vi "UV_Parameters.vi"(6 "A/M (F:auto)":bool, 7 "R/W (F:read)":bool, 8 "error in":errorcluster, 9 "param":T1={"Time_sec"="7005.1", "Head_Pow%"=0, "Temp (C)"=50}, 10 "CHN":T2=255 items=["All"=255, "CH1"=1, "CH2"=2, "CH3"=3, "CH4"=4], 11 "VISA resource":refnum<visa-resource-name>="COM5") -> (0 "error out":errorcluster, 2 "chn param":u8[](array[numeric]) format="%.0x", 3 "VISA resource out":refnum<visa-resource-name>, 5 "Err?":bool)   [LabVIEW 2018]
uses:
  TypeDef/UVLed_channel.ctl
  TypeDef/UVLed_func.ctl
  low_level/convert/LONG_ASCII (SubVI).vi
  low_level/convert/Gen_UV_CMD (SubVI).vi
  low_level/convert/CMD_SUM (SubVI).vi
  low_level/VISA query.vi
panel:
  # "For Manual and Auto Mode Only"
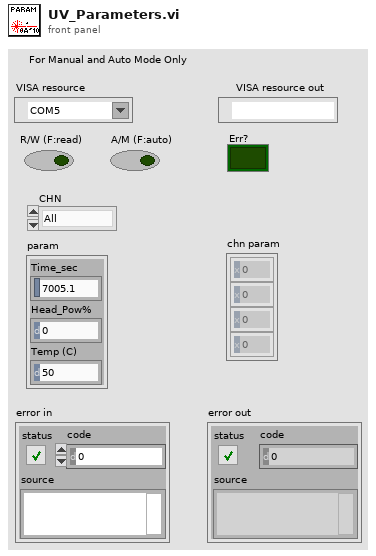
[diagram p1: front panel]
types:
  T1 = cluster{"Time_sec":string, "Head_Pow%":i32, "Temp (C)":u8}
  T2 = typedef "UVLed_channel.ctl" = u16
  T3 = typedef "UVLed_func.ctl" = u16
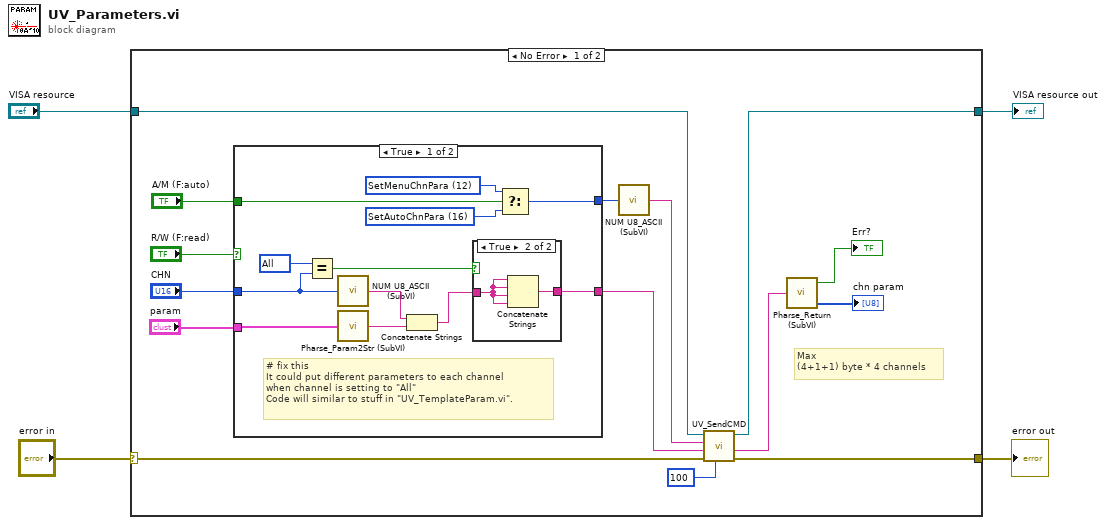
[diagram p0: block diagram]
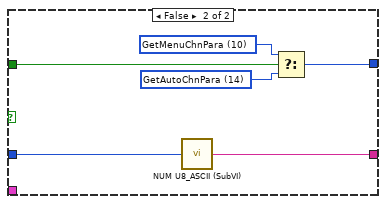
[diagram p3: hidden frame]
diagram:
  n1 = case shown="No Error" "error in" {
    selector: "error in" -> [w16 w42]
    tunnel: [w15 w42] -> w3
    tunnel: "VISA resource" -> [w17 w41]
    tunnel: [w13 w41] -> w1
    frame No Error {
      # "Max\n(4+1+1) byte * 4 channels"
      n2 = case shown="True" "R/W (F:read)" {
        tunnel: [w31 w40] -> w19
        tunnel: "A/M (F:auto)" -> [w30 w37]
        tunnel: [w22 w36] -> w10
        tunnel: "CHN" -> [w26 w35]
        tunnel: "param" -> [w21 _]
        frame True {
          w25 = T2 255 items=["All"=255, "CH1"=1, "CH2"=2, "CH3"=3, "CH4"=4] ("x")
          w28 = T3 16 items=["GetAllStatus"=0, "LightOn"=2, "LightOff"=4, "AllForceOff"=6, "GetMenuChnPara"=10, "SetMenuChnPara"=12, "GetAutoChnPara"=14, "SetAutoChnPara"=16, "GetMenuTemplate"=18, "SetMenuTemplate"=20, "GetAutoTemplate"=22, "SetAutoTemplate"=24, "GetTemplatePara"=26, "SetTemplatePara"=28, "GetMode"=30, "SetMode"=32, "ChkErr"=240] ("Function")
          w29 = T3 12 items=["GetAllStatus"=0, "LightOn"=2, "LightOff"=4, "AllForceOff"=6, "GetMenuChnPara"=10, "SetMenuChnPara"=12, "GetAutoChnPara"=14, "SetAutoChnPara"=16, "GetMenuTemplate"=18, "SetMenuTemplate"=20, "GetAutoTemplate"=22, "SetAutoTemplate"=24, "GetTemplatePara"=26, "SetTemplatePara"=28, "GetMode"=30, "SetMode"=32, "ChkErr"=240] ("Function")
          # "# fix this\nIt could put different parameters to each channel \nwhen channel is setting to \"All\"\nCode will similar to stuff in \"UV_TemplateParam.vi\"."
          n3 = Equal?(x=w25, y=w26) -> (x = y?=w23:bool)
          n4 = call "NUM U8_ASCII (SubVI).vi"("Numeric"=w26) -> ("String out"=w27:string)
          n5 = call "Pharse_Param2Str (SubVI).vi"("param"=w21) -> ("param_cmd"=w20:string)
          n6 = Concatenate Strings(w27, w20) -> (w24:string)
          n7 = case shown="True" w23 {
            tunnel: w24 -> [w32 w34]
            tunnel: [w32 w33] -> w22
            frame False {
            }
            frame True {
              n8 = Concatenate Strings(w34, w34, w34, w34) -> (w33:string)
            }
          }
          n9 = Select(t=w29, s=w30, f=w28) -> (s? t:f=w31:T3)
        }
        frame False {
          w38 = T3 14 items=["GetAllStatus"=0, "LightOn"=2, "LightOff"=4, "AllForceOff"=6, "GetMenuChnPara"=10, "SetMenuChnPara"=12, "GetAutoChnPara"=14, "SetAutoChnPara"=16, "GetMenuTemplate"=18, "SetMenuTemplate"=20, "GetAutoTemplate"=22, "SetAutoTemplate"=24, "GetTemplatePara"=26, "SetTemplatePara"=28, "GetMode"=30, "SetMode"=32, "ChkErr"=240] ("Function")
          w39 = T3 10 items=["GetAllStatus"=0, "LightOn"=2, "LightOff"=4, "AllForceOff"=6, "GetMenuChnPara"=10, "SetMenuChnPara"=12, "GetAutoChnPara"=14, "SetAutoChnPara"=16, "GetMenuTemplate"=18, "SetMenuTemplate"=20, "GetAutoTemplate"=22, "SetAutoTemplate"=24, "GetTemplatePara"=26, "SetTemplatePara"=28, "GetMode"=30, "SetMode"=32, "ChkErr"=240] ("Function")
          n10 = call "NUM U8_ASCII (SubVI).vi"("Numeric"=w35) -> ("String out"=w36:string)
          n11 = Select(t=w39, s=w37, f=w38) -> (s? t:f=w40:T3)
        }
      }
      n12 = call "NUM U8_ASCII (SubVI).vi"("Numeric"=w19) -> ("String out"=w18:string)
      n13 = call "UV_SendCMD.vi"("delay(ms)"=100, "error in"=w16, "value"=w10, "function"=w18, "VISA resource name"=w17) -> ("error out"=w15:errorcluster, "response"=w14:string, "VISA resource name out"=w13:refnum<visa-resource-name>)  [unwired: 4 in]
      n14 = call "Pharse_Return (SubVI).vi"("buffer in"=w14) -> ("byte array"=→"chn param":u8[], "Err?"=→"Err?":bool)  [unwired: 2 in, 1 out]
    }
    frame Error {
    }
  }
  "error out" <- w3
  "VISA resource out" <- w1
